vi "Monitor Setting.vi"(8 "error in (no error)":errorcluster, 9 "Monitor For Gain-Phase (0:Off)":u32(ring) items=["Off", "Rch [V]", "Rch [dBm]", "Rch [dBV]", "Tch [V]", "Tch [dBm]", "Tch [dBV]"], 10 "Monitor For Impedance (0:Off)":u32(ring) items=["Off", "V (AC)", "I (AC) "], 11 "VISA resource name":refnum<visa-resource-name>) -> (0 "error out":errorcluster, 3 "VISA resource name out":refnum<visa-resource-name>)   [LabVIEW 2010, in "Agilent 4194.lvlib"]
doc: "This function sets the impedance and gain-phase monitor function."
uses:
  <instrlib>/Agilent 4194/Agilent 4194.lvlib
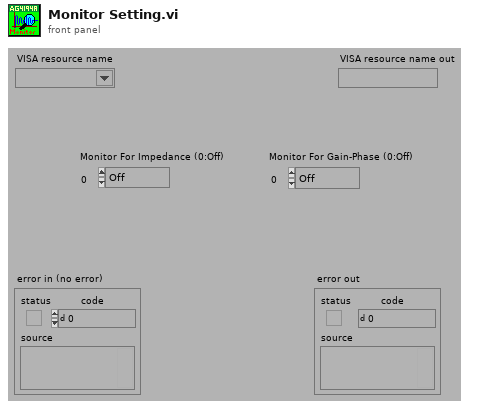
[diagram p1: front panel]
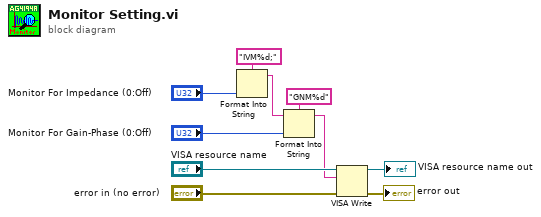
[diagram p0: block diagram]
diagram:
  n1 = Format Into String(format string="IVM%d;", "Monitor For Impedance (0:Off)") -> (resulting string=w9:string)  [unwired: 2 in, 1 out]
  n2 = Format Into String(format string="GNM%d", initial string=w9, "Monitor For Gain-Phase (0:Off)") -> (resulting string=w4:string)  [unwired: 1 in, 1 out]
  n3 = VISA Write(VISA resource name="VISA resource name", write buffer=w4, error in (no error)="error in (no error)") -> (VISA resource name out=→"VISA resource name out":refnum<visa-resource-name>, error out=→"error out":errorcluster)  [unwired: 1 out]
